vi "change tag metadata.vi"(8 "error in":errorcluster, 9 "metadata":string, 10 "tag name":string, 11 "engine configuration in":refnum<class "engine configuration.lvclass">) -> (0 "error out":errorcluster, 3 "engine configuration out":refnum<class "engine configuration.lvclass">)   [LabVIEW 2013, in "engine configuration.lvclass"]
uses:
  engine configuration.lvclass
  <vilib>/NI/Tag Bus/tag/tag descriptor.lvclass
  <vilib>/NI/Tag Bus/tag/tag descriptor.lvclass/tag descriptor.ctl
  engine configuration.lvclass/engine configuration.ctl
  <vilib>/NI/Tag Bus/tag/write tag name.vi
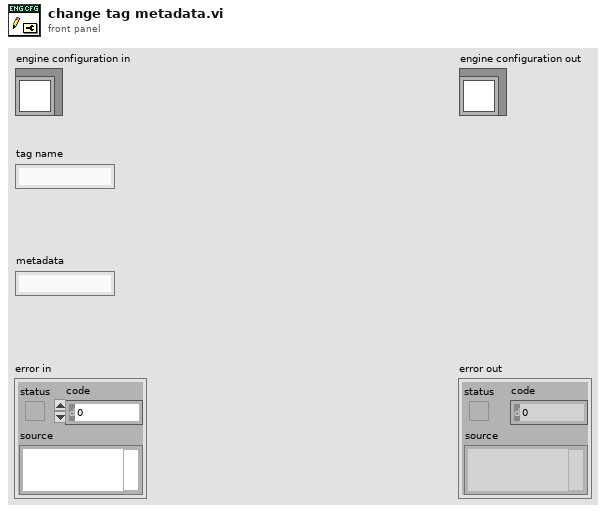
[diagram p1: front panel]
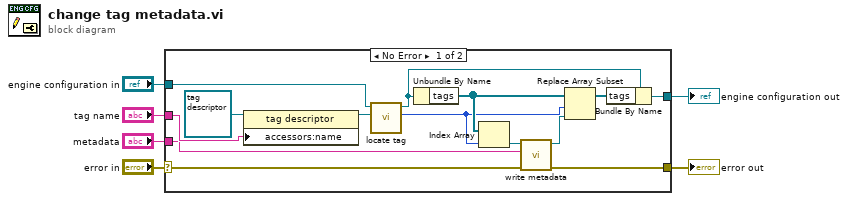
[diagram p0: block diagram]
diagram:
  n1 = case shown="No Error" "error in" {
    selector: "error in" -> [w10 w22]
    tunnel: [w9 w22] -> w5
    tunnel: [w19 w21] -> w3
    tunnel: "engine configuration in" -> [w15 w21]
    tunnel: "tag name" -> [w18 _]
    tunnel: "metadata" -> [w11 _]
    frame No Error {
      n2 = property class="tag descriptor"(reference=refnum<class "tag descriptor.lvclass"> refnum ("tag descriptor"), "accessors:name"=w18) -> (reference out=w12:refnum<class "tag descriptor.lvclass">)  [unwired: 1 in, 1 out]
      n3 = call "locate tag.vi"("tag descriptor"=w12, "engine configuration in"=w15) -> ("index"=w13:i32, "engine configuration out"=w14:refnum<class "engine configuration.lvclass">)  [unwired: 8 in]
      n4 = Unbundle By Name(w14) -> ("tags"=w17:refnum<class "tag descriptor.lvclass">[])
      n5 = Index Array(array=w17, index=w13) -> (element=w7:refnum<class "tag descriptor.lvclass">)
      n6 = call <vilib>:"write metadata.vi"("error in"=w10, "metadata"=w11, "system tag in"=w7) -> ("error out"=w9:errorcluster, "system tag out"=w8:refnum<class "tag descriptor.lvclass">)  [unwired: 7 in]
      n7 = Replace Array Subset(array=w17, new element=w8, index=w13) -> (w16:refnum<class "tag descriptor.lvclass">[])
      n8 = Bundle By Name(cluster=w14, "tags"=w16) -> (w19:refnum<class "engine configuration.lvclass">)
    }
    frame Error {
    }
  }
  "error out" <- w5
  "engine configuration out" <- w3
